vi "Write Piece.vi"(10 "Piece":refnum<class "Piece.lvclass">, 11 "Move in":refnum<class "Move.lvclass">) -> (3 "Move out":refnum<class "Move.lvclass">)   [LabVIEW 2015, in "Chesslib.lvlib" / "Move.lvclass"]
uses:
  Move.lvclass
  Pieces/Piece/Piece.lvclass
  Move.lvclass/Move.ctl
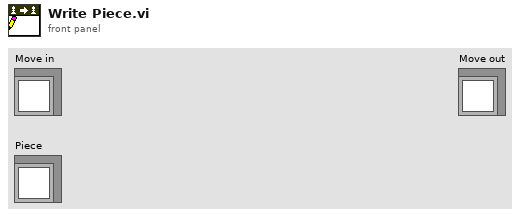
[diagram p1: front panel]
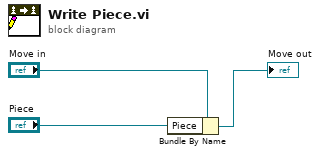
[diagram p0: block diagram]
diagram:
  n1 = Bundle By Name(cluster="Move in", "Piece"="Piece") -> (→"Move out":refnum<class "Move.lvclass">)
